vi "send.vi"(8 "error in (no error)":errorcluster caption="错误输入（无错误）", 10 "send":string, 11 "TCP_client 输入":refnum<class "TCP_client.lvclass">) -> (0 "error out":errorcluster caption="错误输出", 3 "TCP_client 输出":refnum<class "TCP_client.lvclass">)   [LabVIEW 2016, in "数据传输系统-03.lvlib" / "update.lvlib" / "TCP_client.lvclass"]
uses:
  TCP_client.lvclass
  TCP_client.lvclass/TCP_client.ctl
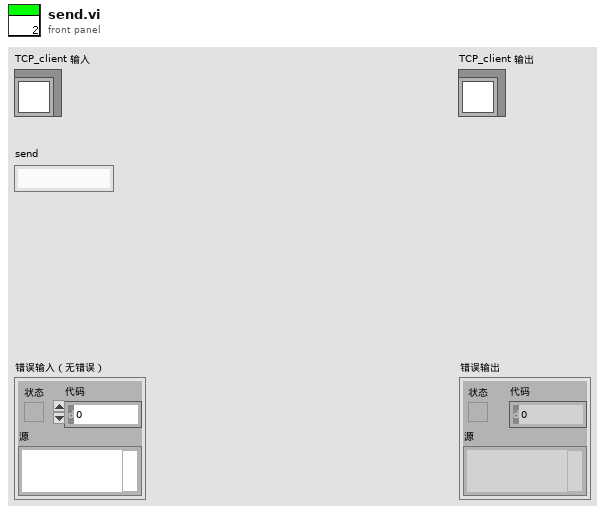
[diagram p1: front panel]
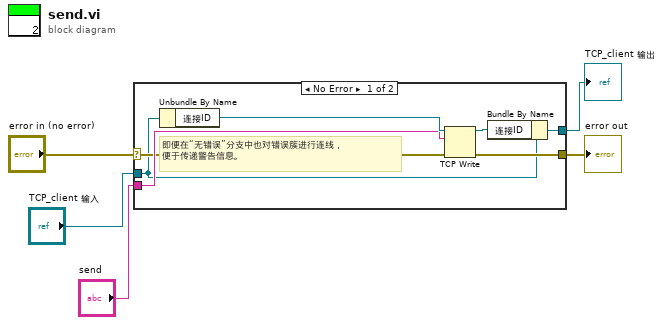
[diagram p0: block diagram]
diagram:
  n1 = case shown="No Error" "error in (no error)" {
    selector: "error in (no error)" -> [w10 w14]
    tunnel: [w9 w14] -> w4
    tunnel: [w6 w13] -> w2
    tunnel: "TCP_client 输入" -> [w8 w13]
    tunnel: "send" -> [w11 _]
    frame No Error {
      # "即便在“无错误”分支中也对错误簇进行连线，\n便于传递警告信息。"
      n2 = Unbundle By Name(w8) -> ("连接ID"=w12:refnum<k5>)
      n3 = TCP Write(connection ID=w12, data in=w11, error in (no error)=w10) -> (connection ID out=w7:refnum<k5>, error out=w9:errorcluster)  [unwired: 1 in, 1 out]
      n4 = Bundle By Name(cluster=w8, "连接ID"=w7) -> (w6:refnum<class "TCP_client.lvclass">)
    }
    frame Error {
    }
  }
  "error out" <- w4
  "TCP_client 输出" <- w2
